vi "DSP_read_fast_sweep.vi"(1 "inst param":T1={"Kind"=12, "Strings"=["Lock-in", "0:12", "V", "X;Y;Sensitivity", "V;V;a.u."], "uint64s"=[5, 19, 3, 0, 0, 0, 0, 0, 0, 27, 12, 2, 2], "Doubles"=[1.0, 0.10000000149011612, 37.70000076293945, 1.0, 0.0, 1000.0, 0.009999999776482582], "DAQmx take out list"=[]}) -> (0 "Data":dbl[][](array[numeric]))   [LabVIEW 2013]
uses:
  SR72xx write-read/SR72XXLV8.llb/SR72XX VISA Write/Read.vi
panel:
  in  "DSP type":u32=7265
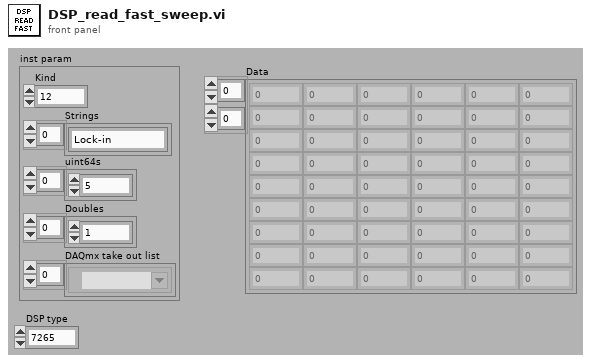
[diagram p1: front panel]
types:
  T1 = cluster{"Kind":u16, "Strings":string[], "uint64s":u64[], "Doubles":dbl[], "DAQmx take out list":refnum<k21>[]}
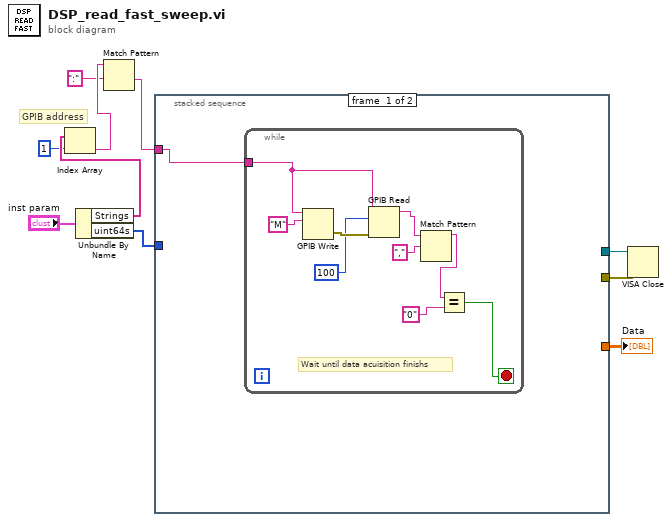
[diagram p0: block diagram]
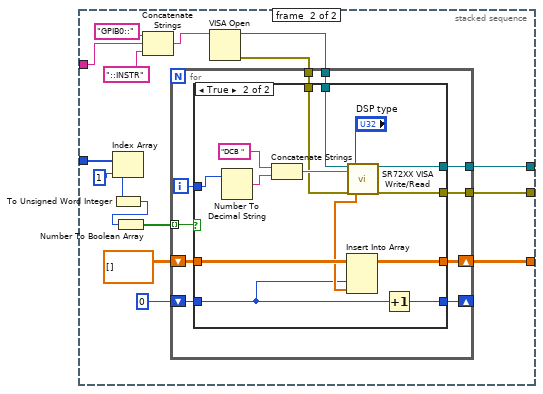
[diagram p2: hidden frame]
diagram:
  # "GPIB address"
  n1 = Unbundle By Name("inst param") -> ("Strings"=w9:string[], "uint64s"=w7:u64[])
  n2 = Index Array(array=w9, index=1) -> (element=w3:string)
  n3 = Match Pattern(string=w3, regular expression=":") -> (after substring=w1:string)  [unwired: 1 in, 3 out]
  n4 = stacked-sequence {
    tunnel: w1 -> [w11 w31]
    tunnel: w7 -> [_ w36]
    tunnel: [_ w25] -> w6
    tunnel: [_ w23] -> w5
    tunnel: [_ w21] -> w4
    frame #0 {
      n5 = while {
        tunnel: w11 -> [w20]
        stop <- w12 stop-if-true
        # "Wait until data acuisition finishs"
        n6 = GPIB Write(0:w20, 1:"M") -> (6:w18:errorcluster)  [unwired: 3 in, 1 out]
        n7 = GPIB Read(0:w20, 1:100, 3:w18) -> (5:w15:string)  [unwired: 2 in, 2 out]
        n8 = Match Pattern(string=w15, regular expression=",") -> (before substring=w13:string)  [unwired: 1 in, 3 out]
        n9 = Equal?(x=w13, y="0") -> (x = y?=w12:bool)
      }
    }
    frame #1 {
      n10 = Index Array(array=w36, index=1) -> (element=w34:u64)
      n11 = To Unsigned Word Integer(number=w34) -> (unsigned 16bit integer=w33:u16)
      n12 = Number To Boolean Array(number=w33) -> (Boolean array=w32:bool[])
      n13 = Concatenate Strings("GPIB0::", w31, "::INSTR") -> (w28:string)
      n14 = VISA Open(VISA resource name=w28) -> (VISA resource name=w27:refnum<visa-resource-name>, error out=w22:errorcluster)  [unwired: 4 in]
      n15 = for {
        tunnel: w32 -> [w46] mode=indexing
        tunnel: w27 -> [w44]
        shift-right: [w43] -> w25
        shift-left: dbl[][] [] -> [w42]
        shift-right: [w40] -> _
        shift-left: 0 -> [w41]
        tunnel: [w39] -> w23
        tunnel: w22 -> [w38]
        tunnel: [w37] -> w21
        i -> [w45]
        n16 = case shown="True" w46 {
          tunnel: w45 -> [_ w64]
          tunnel: w44 -> [w48 w60]
          tunnel: [w50 w58] -> w43
          tunnel: w42 -> [w50 w59]
          tunnel: [w49 w55] -> w40
          tunnel: w41 -> [w49 w56]
          tunnel: [w48 w54] -> w39
          tunnel: w38 -> [w47 w53]
          tunnel: [w47 w52] -> w37
          frame False {
          }
          frame True {
            n17 = Number To Decimal String(number=w64) -> (decimal integer string=w63:string)  [unwired: 1 in]
            n18 = Concatenate Strings("DCB ", w63) -> (w61:string)
            n19 = call "SR72XX VISA Write/Read.vi"("VISA session (for class)"=w60, "Write Command String"=w61, "error in (no error)"=w53, "DSP type"="DSP type") -> ("Array"=w57:dbl[], "VISA session"=w54:refnum<visa-resource-name>, "error out"=w52:errorcluster)  [unwired: 3 in, 10 out]
            n20 = Insert Into Array(array=w59, index (col)=w56, new element=w57) -> (w58:dbl[][])  [unwired: 1 in]
            n21 = Increment(x=w56) -> (x+1=w55:i32)
          }
        }
      }
    }
  }
  "Data" <- w6
  n22 = VISA Close(VISA resource name=w5, error in (no error)=w4) -> ()  [unwired: 1 out]
